vi "M9300A_set_one_ch.vi"(5 "OUT1":bool=TRUE caption="Output1", 7 "AttributeID":u32(ring)=1150009 items=["BACK_PLANE_REFERENCE_ENABLED"=1150015, "BP_OUT_ENABLED"=1150003, "EXTERNAL_REFERENCE_ENABLED"=1150004, "NONVOLATILE_ENABLE_INSTRUMENT_CAL_WARNINGS"=1150029, "NONVOLATILE_ENABLE_MODULE_CAL_WARNINGS"=1150028, "NONVOLATILE_ENABLE_PERIODIC_CAL"=1150027, "OCXO_ENABLED"=1150008, "OUT1_ENABLED"=1150009, "OUT2_ENABLED"=1150010, "OUT3_ENABLED"=1150011, "OUT4_ENABLED"=1150012, "OUT5_ENABLED"=1150013, "PROGRAMMABLE_TRIGGER_ENABLED"=1150033, "REF_10_MHZ_OUT_ENABLED"=1150014, "SIMULATE"=1050005, "TRACE_ENABLED"=1150002], 8 "error in (no error)":errorcluster {"code" format="%.0x"}, 11 "resource string":string="PXI8::0::0::INSTR") -> (0 "error out":errorcluster {"code" format="%.0x"})   [LabVIEW 2021]
uses:
  <instrlib>/Agilent M9300/Agilent M9300.lvlib
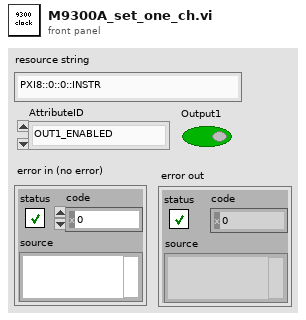
[diagram p1: front panel]
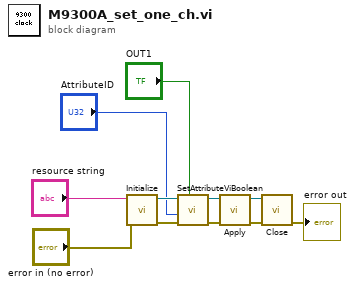
[diagram p0: block diagram]
diagram:
  n1 = call <instrlib>:"Initialize.vi"("error in (no error)"="error in (no error)", "resource string"="resource string") -> ("error out"=w9:errorcluster, "instrument handle out"=w10:refnum<k15>)  [unwired: 8 in]
  n2 = call <instrlib>:"SetAttributeViBoolean.vi"("AttributeValue (Off)"="OUT1", "error in (no error)"=w9, "AttributeID"="AttributeID", "instrument handle"=w10) -> ("error out"=w5:errorcluster, "instrument handle out"=w6:refnum<k15>)  [unwired: 6 in]
  n3 = call <instrlib>:"Apply.vi"("error in (no error)"=w5, "instrument handle"=w6) -> ("error out"=w3:errorcluster, "instrument handle out"=w4:refnum<k15>)  [unwired: 8 in]
  n4 = call <instrlib>:"Close.vi"("error in (no error)"=w3, "instrument handle"=w4) -> ("error out"=→"error out":errorcluster)  [unwired: 9 in]
